vi "blueLocation.vi"() -> (0 "range":string, 1 "pos":string, 2 "Dataout":string="b")   [LabVIEW 2017]
panel:
  out "Image Out":T1(plugin-control)
  out "BLUE":T2
  out "size":i32
  out "convex hull area":dbl
  out "Tayang":dbl
  out "Area":dbl
  out "Height":dbl
  out "Width":dbl
  out "Bottom":dbl
  out "Right":dbl
  out "Up":dbl
  out "Left":dbl
  out "CenterY":dbl
  out "CenterX":dbl
  out "Blue_Data":dbl[](array[numeric])
  out "blue_stop":bool
  out "Numeric":i32
  # "center x"
  # "center y"
  # "left"
  # "up"
  # "right"
  # "bot"
  # "width"
  # "height"
  # "tayang"
  # "area"
  # "convex hull area"
  # "img area"
  # "%area/img area"
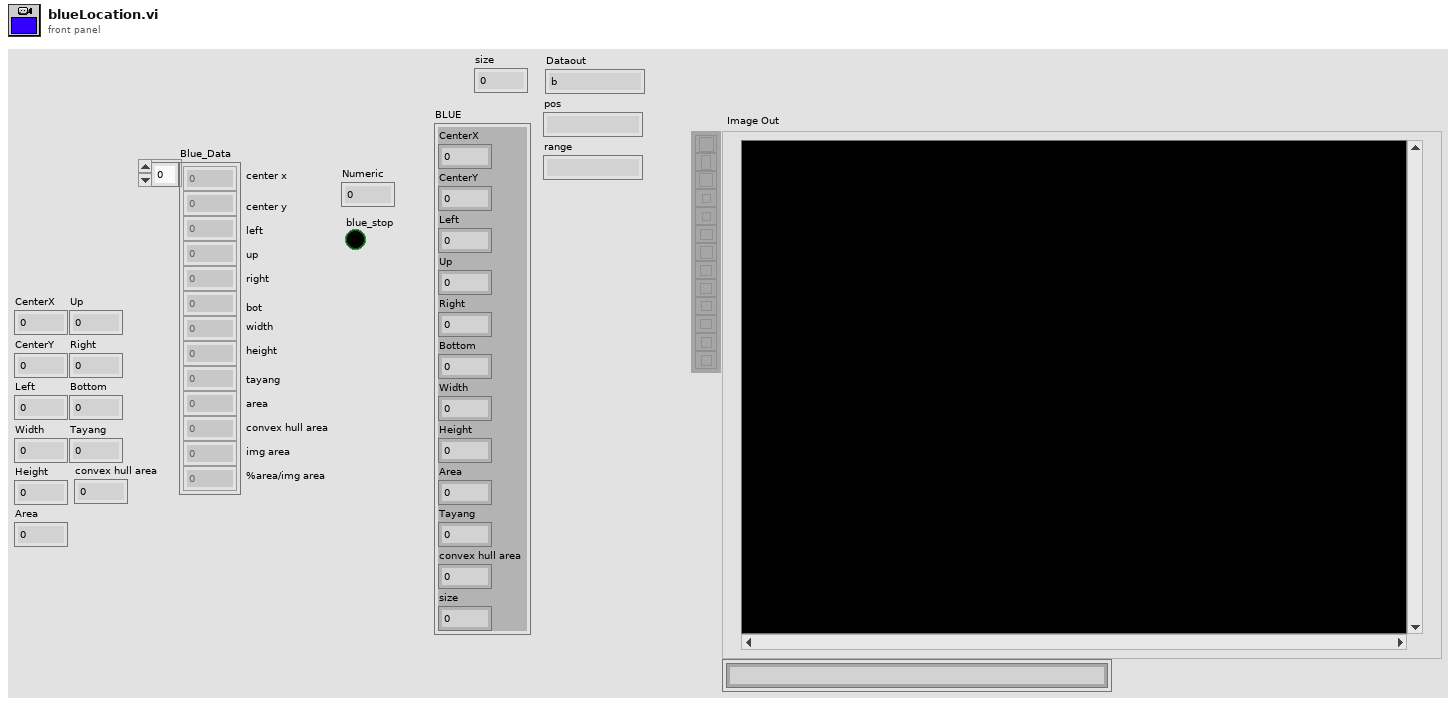
[diagram p1: front panel]
types:
  T1 = typedef "IMAQ Image.ctl" = refnum<image>
  T2 = cluster{"CenterX":dbl, "CenterY":dbl, "Left":dbl, "Up":dbl, "Right":dbl, "Bottom":dbl, "Width":dbl, "Height":dbl, "Area":dbl, "Tayang":dbl, "convex hull area":dbl, "size":i32}
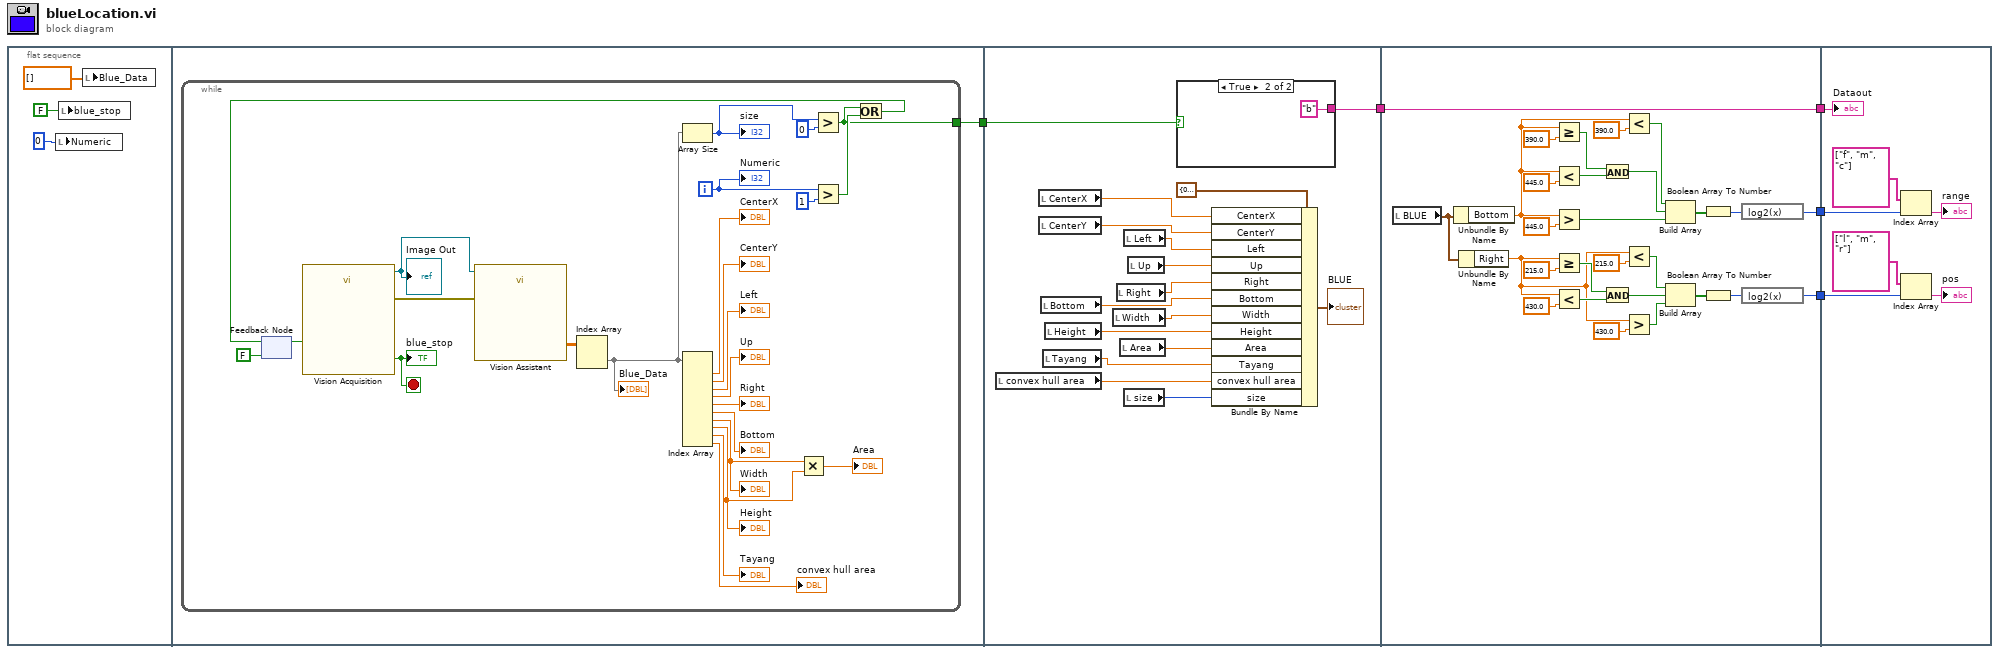
[diagram p0: block diagram]
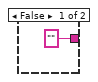
[diagram p2: hidden frame]
diagram:
  n1 = flat-sequence {
    tunnel: [w9] -> w5
    tunnel: w5 -> [w36]
    tunnel: [w35] -> w1
    tunnel: [w68] -> w4
    tunnel: [w56] -> w3
    tunnel: [w53] -> w2
    tunnel: w1 -> [w53]
    tunnel: w4 -> [w86]
    tunnel: w3 -> [w83]
    tunnel: w2 -> [w81]
    frame #0 {
      n2 = local write "Numeric"(0 ("Numeric")) -> ()
      n3 = local write "blue_stop"(FALSE ("blue_stop")) -> ()
      n4 = local write "Blue_Data"(dbl[] [] ("Blue_Data")) -> ()
    }
    frame #1 {
      n5 = while {
        tunnel: [w10] -> w9
        i -> [w29]
        stop <- w24 stop-if-true
        n6 = feedback #1(FALSE) -> (w25:bool)
        n7 = call "Vision Acquisition"("Stop (F)"=w25) -> ("Image Out"=w34:T1, "Stopped"=w24:bool, "error out"=w27:errorcluster)  [unwired: 24 in]
        "blue_stop" <- w24
        "Image Out" <- w34
        n8 = call "Vision Assistant"("Image In"=w34, "error in"=w27) -> ("Particle Measurements (Pixels) (Particle Analysis 1)"=w33:dbl[][])  [unwired: 22 in, 3 out]
        n9 = Index Array(array=w33) -> (element=w11:dbl[])  [unwired: 2 in]
        "Blue_Data" <- w11
        n10 = Array Size(array=w11) -> (size(s)=w32:i32)
        "size" <- w32
        n11 = Index Array(array=w11) -> (element #1=→"CenterX":dbl, element #2=→"CenterY":dbl, element #3=→"Left":dbl, element #4=→"Up":dbl, element #5=→"Right":dbl, element #6=→"Bottom":dbl, element #7=w22:dbl, element #8=w21:dbl, element #9=→"Tayang":dbl, element #10=→"convex hull area":dbl)  [unwired: 10 in]
        "Width" <- w22
        "Height" <- w21
        n12 = Multiply(x=w22, y=w21) -> (x*y=→"Area":dbl)
        n13 = Greater?(x=w32, y=0) -> (0:w10:bool)
        n14 = Greater?(x=w29, y=1) -> (0:w28:bool)
        n15 = Or(x=w10, y=w28) -> (x .or. y?=w26:bool)
        n16 = feedback-in #1(w26) -> ()
        "Numeric" <- w29
      }
    }
    frame #2 {
      n17 = local read "convex hull area"() -> (w40:dbl)
      n18 = local read "CenterX"() -> (w50:dbl)
      n19 = local read "CenterY"() -> (w49:dbl)
      n20 = local read "Bottom"() -> (w45:dbl)
      n21 = local read "Tayang"() -> (w41:dbl)
      n22 = local read "Height"() -> (w43:dbl)
      n23 = local read "Width"() -> (w44:dbl)
      n24 = local read "Right"() -> (w46:dbl)
      n25 = local read "Area"() -> (w42:dbl)
      n26 = local read "Left"() -> (w48:dbl)
      n27 = local read "size"() -> (w38:i32)
      n28 = local read "Up"() -> (w47:dbl)
      n29 = case shown="True" w36 {
        tunnel: ["" "b"] -> w35
        frame False {
        }
        frame True {
        }
      }
      n30 = Bundle By Name(cluster=T2 {"CenterX"=0.0, "CenterY"=0.0, "Left"=0.0, "Up"=0.0, "Right"=0.0, "Bottom"=0.0, "Width"=0.0, "Height"=0.0, "Area"=0.0, "Tayang"=0.0, "convex hull area"=0.0, "size"=0} ("output cluster"), "CenterX"=w50, "CenterY"=w49, "Left"=w48, "Up"=w47, "Right"=w46, "Bottom"=w45, "Width"=w44, "Height"=w43, "Area"=w42, "Tayang"=w41, "convex hull area"=w40, "size"=w38) -> (→"BLUE":T2)
    }
    frame #3 {
      n31 = local read "BLUE"() -> (w80:T2)
      n32 = Unbundle By Name(w80) -> ("Bottom"=w55:dbl)
      n33 = Unbundle By Name(w80) -> ("Right"=w54:dbl)
      n34 = Greater Or Equal?(x=w55, y=390.0) -> (x >= y?=w64:bool)
      n35 = Less?(x=w55, y=445.0) -> (x < y?=w63:bool)
      n36 = Greater?(x=w55, y=445.0) -> (0:w57:bool)
      n37 = Greater Or Equal?(x=w54, y=215.0) -> (x >= y?=w76:bool)
      n38 = Less?(x=w54, y=430.0) -> (x < y?=w75:bool)
      n39 = And(x=w64, y=w63) -> (x .and. y?=w58:bool)
      n40 = And(x=w76, y=w75) -> (x .and. y?=w72:bool)
      n41 = Less?(x=w55, y=390.0) -> (x < y?=w59:bool)
      n42 = Less?(x=w54, y=215.0) -> (x < y?=w73:bool)
      n43 = Greater?(x=w54, y=430.0) -> (0:w71:bool)
      n44 = Build Array(w59, w58, w57) -> (w61:bool[])
      n45 = Build Array(w73, w72, w71) -> (w70:bool[])
      n46 = Boolean Array To Number(Boolean array=w61) -> (number=w60:u32)
      n47 = Boolean Array To Number(Boolean array=w70) -> (number=w69:u32)
      n48 = expression code="log2(x)"(w60) -> (w56:u32)
      n49 = expression code="log2(x)"(w69) -> (w68:u32)
    }
    frame #4 {
      n50 = Index Array(array=string[] ["f", "m", "c"], index=w83) -> (element=→"range":string)
      n51 = Index Array(array=string[] ["l", "m", "r"], index=w86) -> (element=→"pos":string)
      "Dataout" <- w81
    }
  }
